vi "ActorCoreEvent.vi"(8 "error in (no error)":errorcluster, 10 "ActorCoreMessage":string, 11 "SoftwareSetup in":refnum<class "SoftwareSetup.lvclass">) -> (0 "error out":errorcluster, 3 "SoftwareSetup out":refnum<class "SoftwareSetup.lvclass">)   [LabVIEW 2019, in "SoftwareSetup.lvlib" / "SoftwareSetup.lvclass"]
uses:
  SoftwareSetup.lvclass
  SoftwareSetup.lvclass/SoftwareSetup.ctl
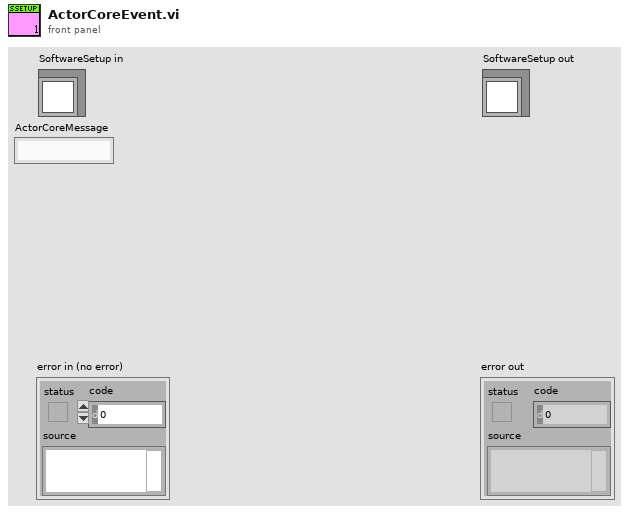
[diagram p1: front panel]
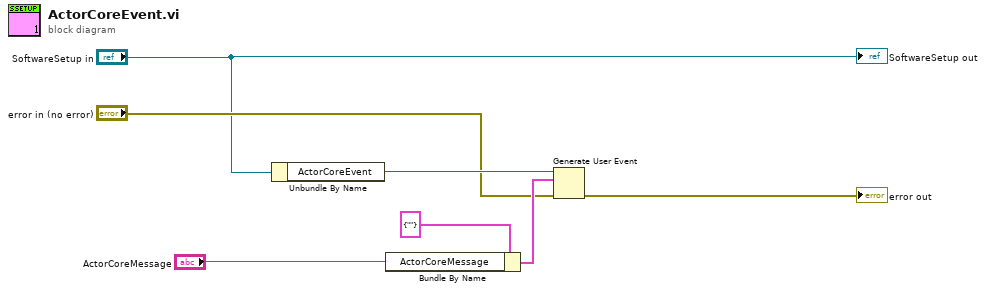
[diagram p0: block diagram]
diagram:
  n1 = Unbundle By Name("SoftwareSetup in") -> ("ActorCoreEvent"=w7:refnum<user-event>)
  n2 = Bundle By Name(cluster=cluster{"ActorCoreMessage":string} {"ActorCoreMessage"=""} ("event data"), "ActorCoreMessage"="ActorCoreMessage") -> (w5:cluster{"ActorCoreMessage":string})
  n3 = Generate User Event(user event=w7, event data cluster=w5, error in="error in (no error)") -> (error out=→"error out":errorcluster)  [unwired: 1 in, 1 out]
  "SoftwareSetup out" <- "SoftwareSetup in"
